vi "Two Sensor Monitor.vi"() -> ()   [LabVIEW 2021]
uses:
  <vilib>/Utility/file.llb/Write Delimited Spreadsheet (DBL).vi
panel:
  in  "Override (0 to override)":dbl
  in  "CONFIGURATION CLUSTER OVERRIDE":T1
  out "Fixed/Auto Range":dbl
  out "Temperature Sensor":u32
  out "millisecond timer value":u32
  out "CONFIGURATION CLUSTER":T1
  out "RESISTANCE (OHMS)":sgl
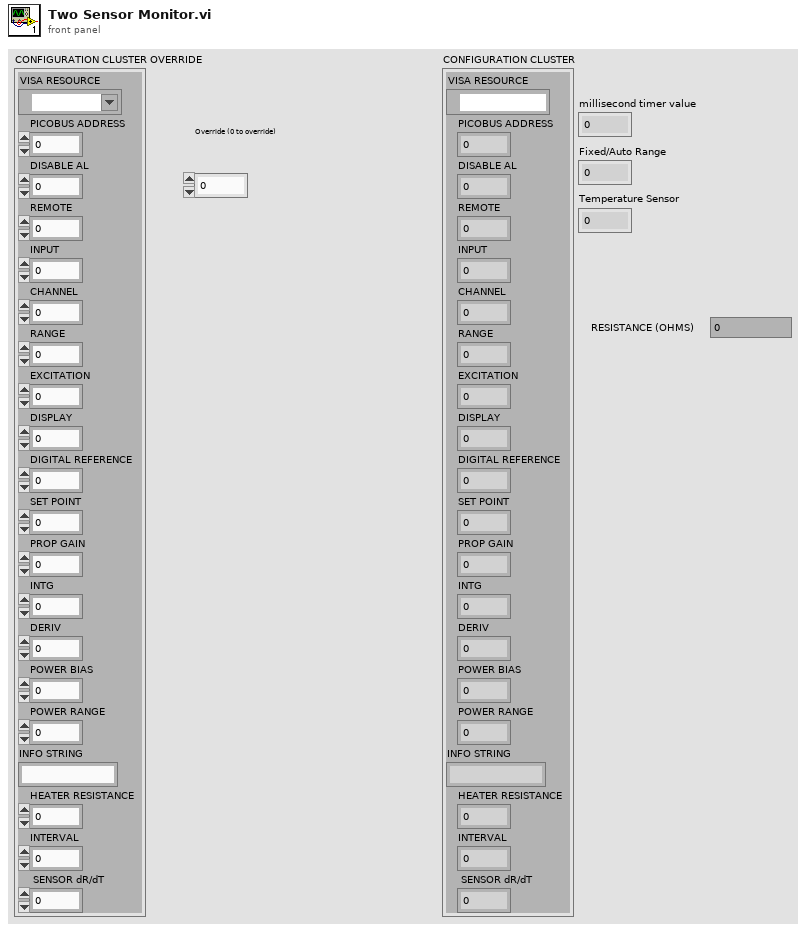
[diagram p1: front panel]
types:
  T1 = cluster{"VISA RESOURCE":refnum<visa-resource-name>, "PICOBUS ADDRESS":u8, "DISABLE AL":u8, "REMOTE":u8, "INPUT":u8, "CHANNEL":u8, "RANGE":u8, "EXCITATION":u8, "DISPLAY":u8, "DIGITAL REFERENCE":u16, "SET POINT":dbl, "PROP GAIN":u8, "INTG":u8, "DERIV":u8, "POWER BIAS":u8, "POWER RANGE":u8, "INFO STRING":string, "HEATER RESISTANCE":dbl, "INTERVAL":u8, " SENSOR dR/dT":u8}
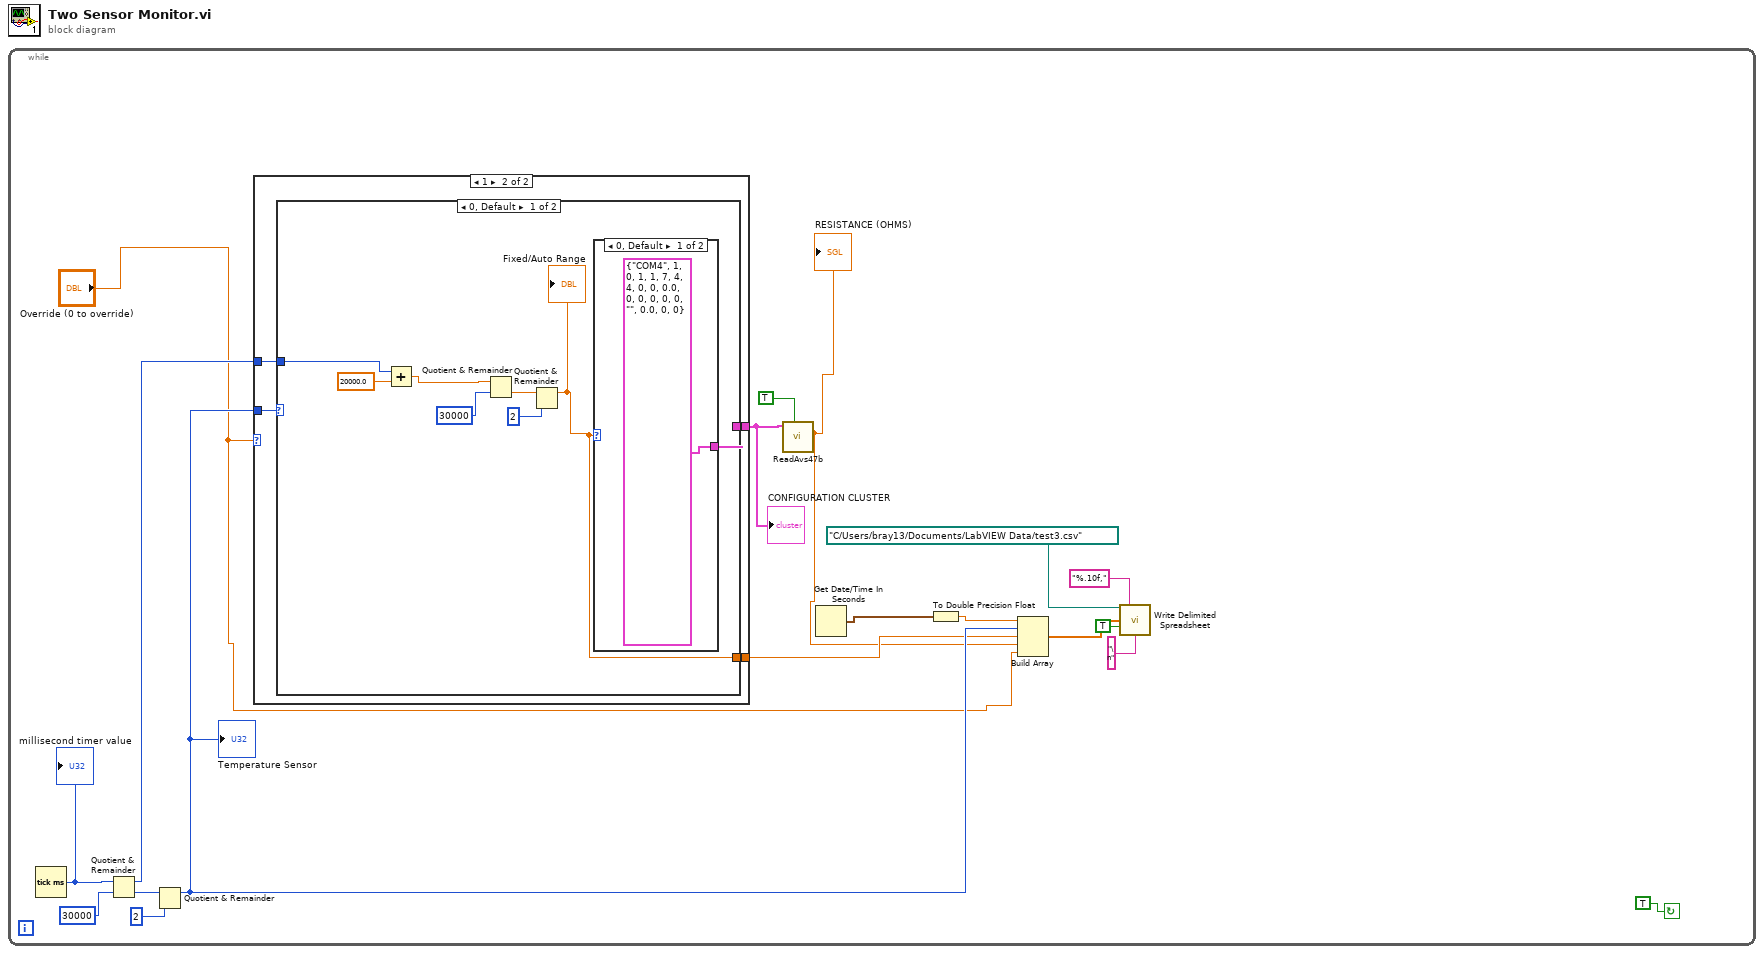
[diagram p0: block diagram]
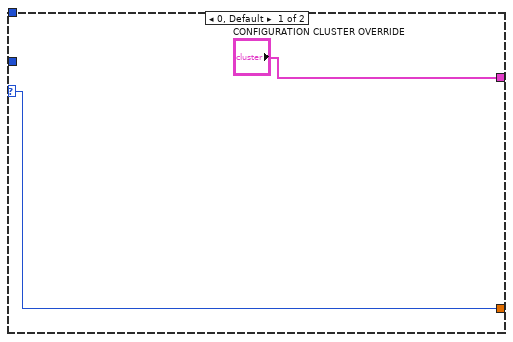
[diagram p2: hidden frame]
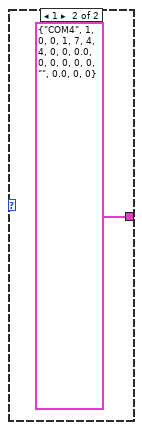
[diagram p3: hidden frame]
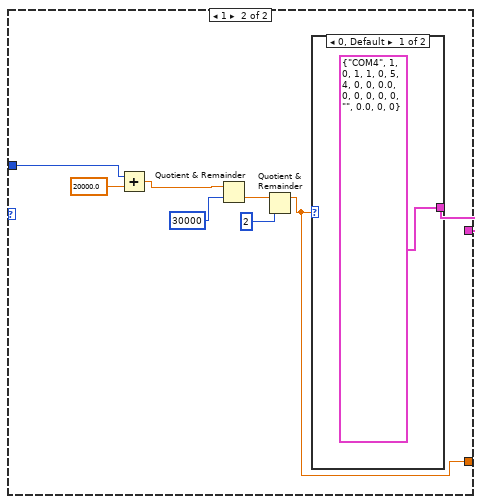
[diagram p4: hidden frame]
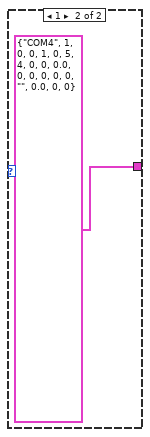
[diagram p5: hidden frame]
diagram:
  n1 = while {
    stop <- TRUE continue-if-true
    n2 = Tick Count (ms)() -> (millisecond timer value=w14:u32)
    "millisecond timer value" <- w14
    n3 = Quotient & Remainder(x=w14, y=u32 30000) -> (x-y*floor(x/y)=w12:u32, floor(x/y)=w17:u32)
    n4 = Quotient & Remainder(x=w17, y=u32 2) -> (x-y*floor(x/y)=w9:u32)  [unwired: 1 out]
    "Temperature Sensor" <- w9
    n5 = case shown="1" "Override (0 to override)" {
      selector: "Override (0 to override)" -> [w20 _]
      tunnel: ["CONFIGURATION CLUSTER OVERRIDE" w25] -> w13
      tunnel: w12 -> [_ w24]
      tunnel: w9 -> [_ w23]
      tunnel: [w20 w22] -> w8
      frame 0, Default {
      }
      frame 1 {
        n6 = case shown="0, Default" w23 {
          tunnel: w24 -> [w28 w38]
          tunnel: [w27 w37] -> w25
          tunnel: [w26 w36] -> w22
          frame 0, Default {
            n7 = Add(x=w28, y=20000.0) -> (x+y=w30:dbl)
            n8 = Quotient & Remainder(x=w30, y=u32 30000) -> (floor(x/y)=w32:dbl)  [unwired: 1 out]
            n9 = Quotient & Remainder(x=w32, y=u32 2) -> (x-y*floor(x/y)=w26:dbl)  [unwired: 1 out]
            "Fixed/Auto Range" <- w26
            n10 = case shown="0, Default" w26 {
              tunnel: [T1 {"VISA RESOURCE"="COM4", "PICOBUS ADDRESS"=1, "DISABLE AL"=0, "REMOTE"=1, "INPUT"=1, "CHANNEL"=7, "RANGE"=4, "EXCITATION"=4, "DISPLAY"=0, "DIGITAL REFERENCE"=0, "SET POINT"=0.0, "PROP GAIN"=0, "INTG"=0, "DERIV"=0, "POWER BIAS"=0, "POWER RANGE"=0, "INFO STRING"="", "HEATER RESISTANCE"=0.0, "INTERVAL"=0, " SENSOR dR/dT"=0} ("CONFIGURATION CLUSTER") T1 {"VISA RESOURCE"="COM4", "PICOBUS ADDRESS"=1, "DISABLE AL"=0, "REMOTE"=0, "INPUT"=1, "CHANNEL"=7, "RANGE"=4, "EXCITATION"=4, "DISPLAY"=0, "DIGITAL REFERENCE"=0, "SET POINT"=0.0, "PROP GAIN"=0, "INTG"=0, "DERIV"=0, "POWER BIAS"=0, "POWER RANGE"=0, "INFO STRING"="", "HEATER RESISTANCE"=0.0, "INTERVAL"=0, " SENSOR dR/dT"=0} ("CONFIGURATION CLUSTER")] -> w27
              frame 0, Default {
              }
              frame 1 {
              }
            }
          }
          frame 1 {
            n11 = Add(x=w38, y=20000.0) -> (x+y=w40:dbl)
            n12 = Quotient & Remainder(x=w40, y=u32 30000) -> (floor(x/y)=w42:dbl)  [unwired: 1 out]
            n13 = Quotient & Remainder(x=w42, y=u32 2) -> (x-y*floor(x/y)=w36:dbl)  [unwired: 1 out]
            n14 = case shown="0, Default" w36 {
              tunnel: [T1 {"VISA RESOURCE"="COM4", "PICOBUS ADDRESS"=1, "DISABLE AL"=0, "REMOTE"=1, "INPUT"=1, "CHANNEL"=0, "RANGE"=5, "EXCITATION"=4, "DISPLAY"=0, "DIGITAL REFERENCE"=0, "SET POINT"=0.0, "PROP GAIN"=0, "INTG"=0, "DERIV"=0, "POWER BIAS"=0, "POWER RANGE"=0, "INFO STRING"="", "HEATER RESISTANCE"=0.0, "INTERVAL"=0, " SENSOR dR/dT"=0} ("CONFIGURATION CLUSTER") T1 {"VISA RESOURCE"="COM4", "PICOBUS ADDRESS"=1, "DISABLE AL"=0, "REMOTE"=0, "INPUT"=1, "CHANNEL"=0, "RANGE"=5, "EXCITATION"=4, "DISPLAY"=0, "DIGITAL REFERENCE"=0, "SET POINT"=0.0, "PROP GAIN"=0, "INTG"=0, "DERIV"=0, "POWER BIAS"=0, "POWER RANGE"=0, "INFO STRING"="", "HEATER RESISTANCE"=0.0, "INTERVAL"=0, " SENSOR dR/dT"=0} ("CONFIGURATION CLUSTER")] -> w37
              frame 0, Default {
              }
              frame 1 {
              }
            }
          }
        }
      }
    }
    "CONFIGURATION CLUSTER" <- w13
    n15 = call "ReadAvs47b.vi"("SYNCHRONISE TO ADC"=TRUE, "CONFIGURATION CLUSTER"=w13) -> ("RESISTANCE (OHMS)"=w7:sgl)  [unwired: 4 in, 5 out]
    "RESISTANCE (OHMS)" <- w7
    n16 = Get Date/Time In Seconds() -> (seconds since 1Jan1904=w11:timestamp)
    n17 = To Double Precision Float(number=w11) -> (double precision float=w10:dbl)
    n18 = Build Array(w10, w9, w8, w7, "Override (0 to override)") -> (w6:dbl[])
    n19 = call-poly <vilib>:"Write Delimited Spreadsheet.vi"("file path (dialog if empty)"=path "C:/Users/bray13/Documents/LabVIEW Data/test3.csv", "format (%.3f)"="%.10f,", "1D data"=w6, "append to file? (new file:F)"=TRUE, "delimiter (\\t)"="\n" ("delimiter (\\t)")) -> ()  [unwired: 9 in, 2 out]
  }
